vi "Calculate Zoom From Mouse Wheel.vi"(8 "Image Center Position":cluster{"X":u32, "Y":u32}={"X"=2, "Y"=2}, 9 "Last Mouse Position":cluster{"X":i32, "Y":i32}={"X"=2, "Y"=2}, 10 "Current Zoom Factor":sgl format="%#_13g", 11 "Delta":i32) -> (2 "New Center Position":cluster{dbl, dbl}, 3 "New Zoom":cluster{dbl, dbl})   [LabVIEW 2021, in "Image.lvlib"]
uses:
  Image.lvlib
  <vilib>/vision/NI_Vision_Development_Module.lvlib
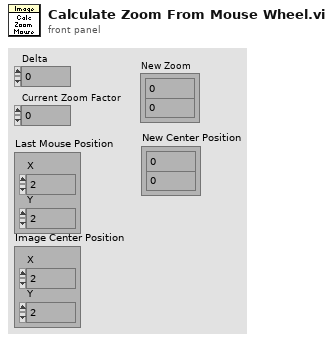
[diagram p1: front panel]
types:
  T1 = cluster{"Current Zoom Factor":dbl, "Current Zoom Factor":dbl}
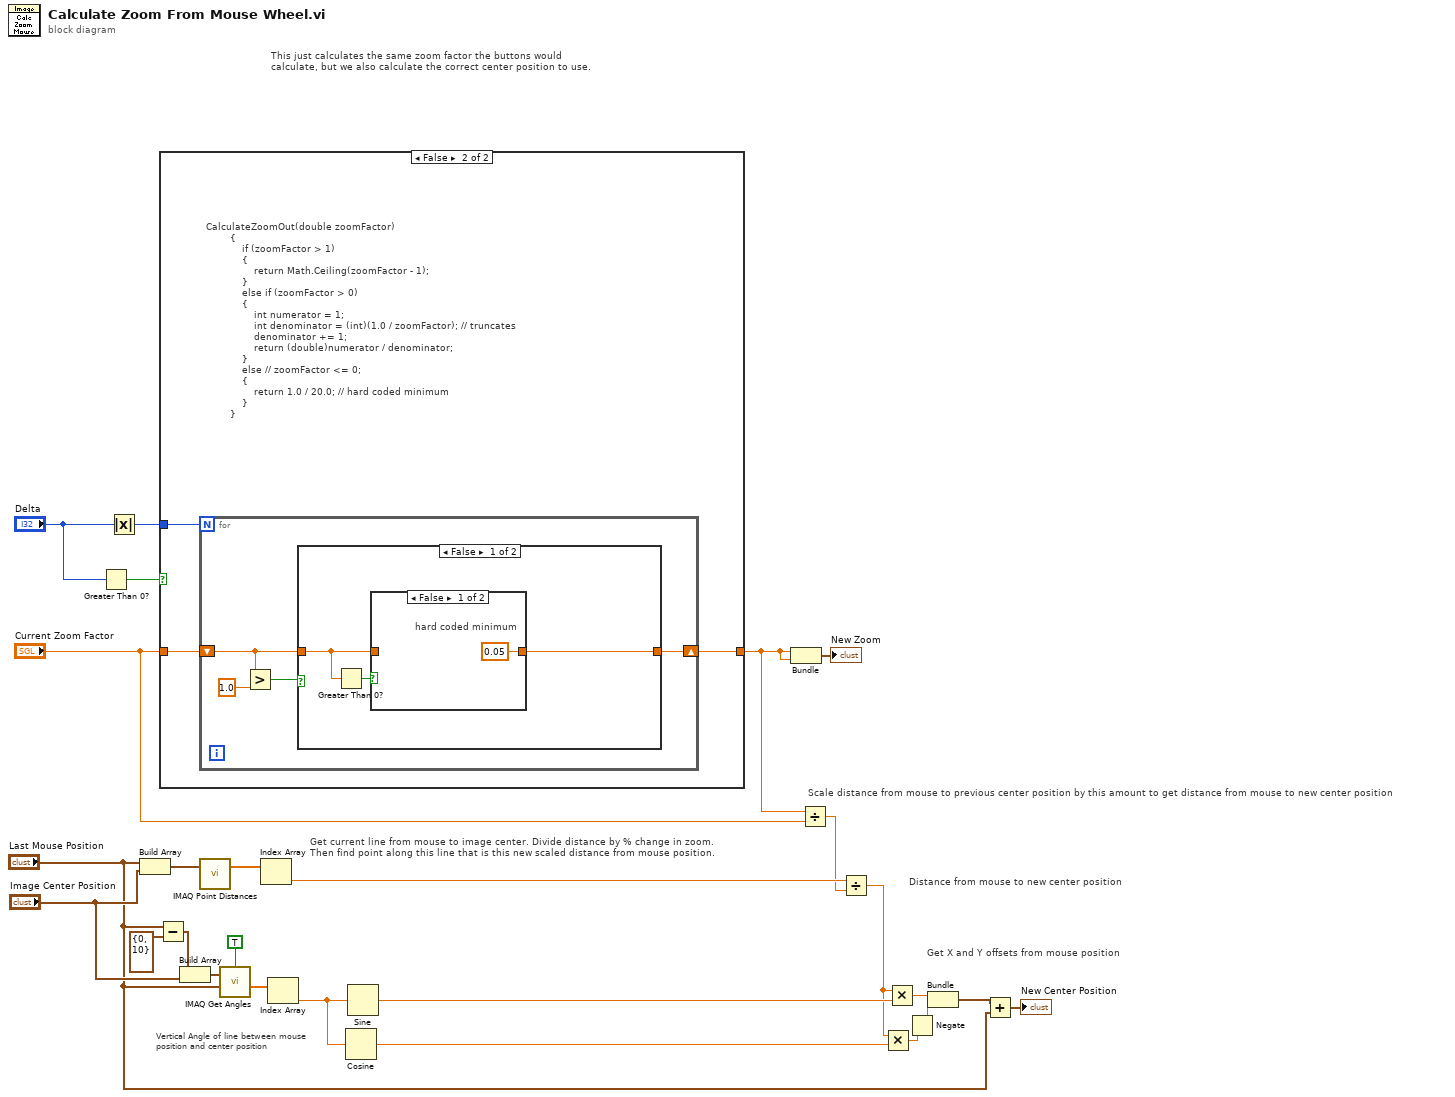
[diagram p0: block diagram]
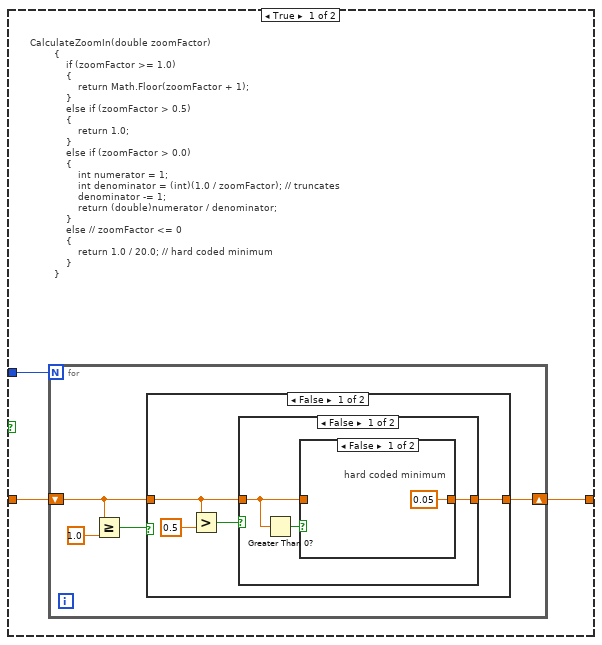
[diagram p2: hidden frame]
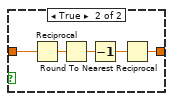
[diagram p3: hidden frame]
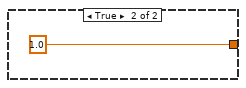
[diagram p4: hidden frame]
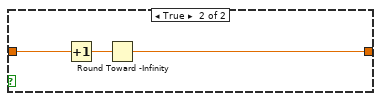
[diagram p5: hidden frame]
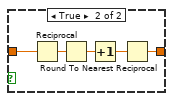
[diagram p6: hidden frame]
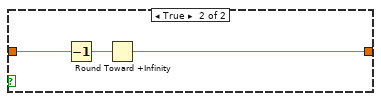
[diagram p7: hidden frame]
diagram:
  # "This just calculates the same zoom factor the buttons would calculate, but we also calculate the correct center position to use."
  # "Get X and Y offsets from mouse position"
  # "Vertical Angle of line between mouse position and center position"
  # "Get current line from mouse to image center. Divide distance by % change in zoom. Then find point along this line that is this new scaled distance from mouse position."
  # "Distance from mouse to new center position"
  # "Scale distance from mouse to previous center position by this amount to get distance from mouse to new center position"
  n1 = Greater Than 0?(x="Delta") -> (x > 0?=w23:bool)
  n2 = Absolute Value(x="Delta") -> (abs(x)=w24:i32)
  n3 = Build Array("Last Mouse Position", "Image Center Position") -> (w17:cluster{"X":u32, "Y":u32}[])
  n4 = Subtract(x="Last Mouse Position", y=cluster{"X":i32, "Y":i32} {"X"=0, "Y"=10}) -> (x-y=w14:cluster{"X":i32, "Y":i32})
  n5 = case shown="False" w23 {
    tunnel: "Current Zoom Factor" -> [w29 w53]
    tunnel: [w28 w52] -> w22
    tunnel: w24 -> [w27 w51]
    frame True {
      # "CalculateZoomIn(double zoomFactor)\n        {\n            if (zoomFactor >= 1.0)\n            {\n                return Math.Floor(zoomFactor + 1);\n            }\n            else if (zoomFactor > 0.5)\n            {\n                return 1.0;\n            }\n            else if (zoomFactor > 0.0)\n            {\n                int numerator = 1;\n                int denominator = (int)(1.0 / zoomFactor); // truncates\n                denominator -= 1;\n                return (double)numerator / denominator;\n            }\n            else // zoomFactor <= 0\n            {\n                return 1.0 / 20.0; // hard coded minimum\n            }\n        }"
      n6 = for {
        N: w27 -> [_]
        shift-right: [w30] -> w28
        shift-left: w29 -> [w31]
        n7 = Greater Or Equal?(x=w31, y=1.0) -> (x >= y?=w32:bool)
        n8 = case shown="False" w32 {
          tunnel: w31 -> [w34 w50]
          tunnel: [w35 w48] -> w30
          frame False {
            n9 = Greater?(x=w34, y=0.5) -> (0:w36:bool)
            n10 = case shown="False" w36 {
              tunnel: [w38 1.0] -> w35
              tunnel: w34 -> [w39 _]
              frame False {
                n11 = Greater Than 0?(x=w39) -> (x > 0?=w40:bool)
                n12 = case shown="False" w40 {
                  tunnel: w39 -> [_ w46]
                  tunnel: [0.05 w42] -> w38
                  frame False {
                    # "hard coded minimum"
                  }
                  frame True {
                    n13 = Reciprocal(x=w46) -> (1/x=w45:dbl)
                    n14 = Round To Nearest(number=w45) -> (nearest integer value=w44:dbl)
                    n15 = Decrement(x=w44) -> (x-1=w43:dbl)
                    n16 = Reciprocal(x=w43) -> (1/x=w42:dbl)
                  }
                }
              }
              frame True {
              }
            }
          }
          frame True {
            n17 = Increment(x=w50) -> (x+1=w49:dbl)
            n18 = Round Toward -Infinity(1:w49) -> (0:w48:dbl)
          }
        }
      }
    }
    frame False {
      # "CalculateZoomOut(double zoomFactor)\n        {\n            if (zoomFactor > 1)\n            {\n                return Math.Ceiling(zoomFactor - 1);\n            }\n            else if (zoomFactor > 0)\n            {\n                int numerator = 1;\n                int denominator = (int)(1.0 / zoomFactor); // truncates\n                denominator += 1;\n                return (double)numerator / denominator;\n            }\n            else // zoomFactor <= 0;\n            {\n                return 1.0 / 20.0; // hard coded minimum\n            }\n        }"
      n19 = for {
        N: w51 -> [_]
        shift-right: [w54] -> w52
        shift-left: w53 -> [w55]
        n20 = Greater?(x=w55, y=1.0) -> (0:w56:bool)
        n21 = case shown="False" w56 {
          tunnel: w55 -> [w59 w69]
          tunnel: [w60 w67] -> w54
          frame False {
            n22 = Greater Than 0?(x=w59) -> (x > 0?=w58:bool)
            n23 = case shown="False" w58 {
              tunnel: w59 -> [_ w66]
              tunnel: [0.05 w62] -> w60
              frame False {
                # "hard coded minimum"
              }
              frame True {
                n24 = Reciprocal(x=w66) -> (1/x=w65:dbl)
                n25 = Round To Nearest(number=w65) -> (nearest integer value=w64:dbl)
                n26 = Increment(x=w64) -> (x+1=w63:dbl)
                n27 = Reciprocal(x=w63) -> (1/x=w62:dbl)
              }
            }
          }
          frame True {
            n28 = Decrement(x=w69) -> (x-1=w68:dbl)
            n29 = Round Toward +Infinity(x=w68) -> (ceil(x): smallest int >= x=w67:dbl)
          }
        }
      }
    }
  }
  n30 = Build Array(w14, "Image Center Position") -> (w12:cluster{"X":u32, "Y":u32}[])
  n31 = call "IMAQ Point Distances"("Points"=w17) -> ("Distances"=w20:sgl[])  [unwired: 4 in, 1 out]
  n32 = call "IMAQ Get Angles"("Vertex"="Last Mouse Position", "Points"=w12, "Use Vertex (No)"=TRUE) -> ("Angles (rad)"=w11:sgl[])  [unwired: 2 in, 2 out]
  n33 = Index Array(array=w20) -> (element=w19:sgl)  [unwired: 1 in]
  n34 = Index Array(array=w11) -> (element=w1:sgl)  [unwired: 1 in]
  n35 = Cosine(x=w1) -> (cos(x)=w9:sgl)
  n36 = Sine(x=w1) -> (sin(x)=w10:sgl)
  n37 = Bundle("Current Zoom Factor"=w22, "Current Zoom Factor"=w22) -> (→"New Zoom":T1)  [unwired: 1 in]
  n38 = Divide(x=w22, y="Current Zoom Factor") -> (x/y=w18:dbl)
  n39 = Divide(x=w19, y=w18) -> (x/y=w2:dbl)
  n40 = Multiply(x=w2, y=w9) -> (x*y=w7:dbl)
  n41 = Multiply(x=w2, y=w10) -> (x*y=w8:dbl)
  n42 = Negate(x=w7) -> (-x=w4:dbl)
  n43 = Bundle(w8, w4) -> (w6:cluster{dbl, dbl})  [unwired: 1 in]
  n44 = Add(x=w6, y="Last Mouse Position") -> (x+y=→"New Center Position":cluster{dbl, dbl})
